vi "Integral.vi"(0 "KIT-QA in":refnum<class "KIT-QA.lvclass">, 1 "-t1":dbl[unit], 2 "t100":dbl[unit], 5 "error in (no error)":errorcluster) -> (14 "KIT-QA out":refnum<class "KIT-QA.lvclass">, 15 "Integral":dbl, 17 "Temperature":dbl, 18 "DCCT@-t1":dbl format="%0.2f", 19 "error out":errorcluster)   [LabVIEW 2015, in "KIT-QA.lvlib" / "KIT-QA.lvclass"]
doc: "Piotr's Integral"
uses:
  KIT-QA.lvclass
  KIT-QA.lvclass/KIT-QA.ctl
  <vilib>/Waveform/WDTOps.llb/WDT Get Waveform Subset DBL.vi
  <vilib>/Waveform/WDTOps.llb/WDT Get XY Value DBL.vi
  <vilib>/Analysis/NI_AALPro.lvlib
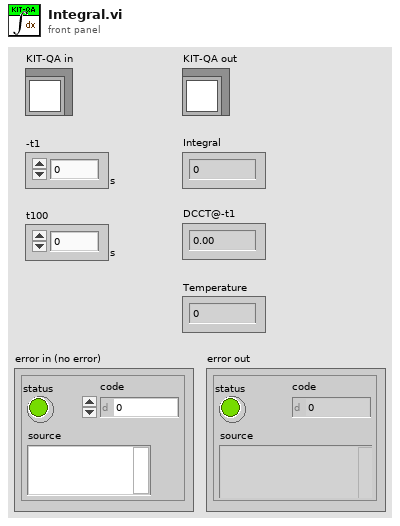
[diagram p1: front panel]
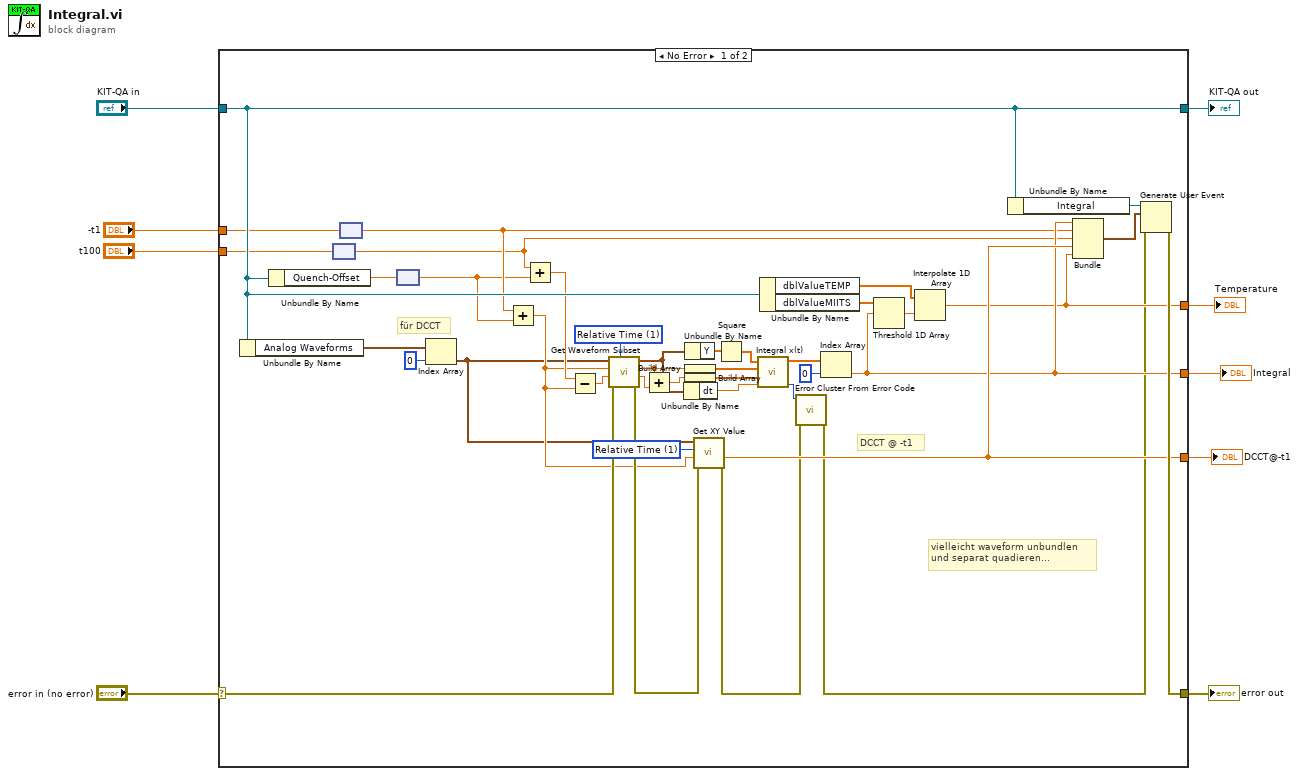
[diagram p0: block diagram]
diagram:
  n1 = case shown="No Error" "error in (no error)" {
    selector: "error in (no error)" -> [w47 w51]
    tunnel: [w49 w51] -> w8
    tunnel: [w31 w50] -> w6
    tunnel: "KIT-QA in" -> [w31 w50]
    tunnel: [w33 _] -> w5
    tunnel: "-t1" -> [w28 _]
    tunnel: "t100" -> [w26 _]
    tunnel: [w41 _] -> w2
    tunnel: [w32 _] -> w1
    frame No Error {
      w10 = u16 1 items=["Samples", "Relative Time"] ("start/duration format")
      w43 = u16 1 items=["Samples", "Relative Time"] ("Y position format")
      # "vielleicht waveform unbundlen\nund separat quadieren..."
      # "DCCT @ -t1"
      # "für DCCT"
      n2 = Unbundle By Name(w31) -> ("Analog Waveforms"=w37:waveform(dbl)[])
      n3 = Unbundle By Name(w31) -> ("Quench-Offset"=w24:dbl[unit])
      n4 = node(w26) -> (w25:dbl)
      n5 = node(w28) -> (w27:dbl)
      n6 = node(w24) -> (w23:dbl)
      n7 = Index Array(array=w37, index=0) -> (element=w17:waveform(dbl))
      n8 = Add(x=w27, y=w23) -> (x+y=w29:dbl)
      n9 = Add(x=w25, y=w23) -> (x+y=w30:dbl)
      n10 = Subtract(x=w30, y=w29) -> (x-y=w39:dbl)
      n11 = call-poly <vilib>:"Get Waveform Subset.vi"("start/duration format"=w10, "error in (no error)"=w47, "duration"=w39, "start samples/time"=w29, "waveform in"=w17) -> ("error out"=w42:errorcluster, "actual duration"=w14:dbl, "actual start samples/time"=w13:dbl, "waveform out"=w16:waveform(dbl))  [unwired: 1 in]
      n12 = Add(x=w13, y=w14) -> (x+y=w12:dbl)
      n13 = Unbundle By Name(w16) -> ("dt"=w44:dbl)
      n14 = Unbundle By Name(w16) -> ("Y"=w19:dbl[])
      n15 = Build Array(w13) -> (w15:dbl[])
      n16 = Build Array(w12) -> (w11:dbl[])
      n17 = call-poly <vilib>:"Get XY Value.vi"("error in (no error)"=w42, "Y position"=w29, "Y position format"=w43, "waveform in"=w17) -> ("error out"=w21:errorcluster, "Y value"=w41:dbl)  [unwired: 3 in, 3 out]
      n18 = Square(x=w19) -> (x^2=w18:dbl[])
      n19 = call <vilib>:"Integral x(t).vi"("dt"=w44, "Final Condition"=w11, "Initial Condition"=w15, "X"=w18) -> ("error"=w22:i32, "Integral X"=w46:dbl[])  [unwired: 6 in]
      n20 = Unbundle By Name(w31) -> ("dblValueTEMP"=w35:dbl[], "dblValueMIITS"=w34:dbl[])
      n21 = call <vilib>:"Error Cluster From Error Code.vi"("error in (no error)"=w21, "error code (0)"=w22) -> ("error out"=w20:errorcluster)  [unwired: 7 in]
      n22 = Index Array(array=w46, index=0) -> (element=w33:dbl)
      n23 = Threshold 1D Array(2:w33, 3:w34) -> (0:w36:dbl)  [unwired: 1 in]
      n24 = Interpolate 1D Array(1:w36, 2:w35) -> (0:w32:dbl)
      n25 = Unbundle By Name(w31) -> ("Integral"=w40:refnum<user-event>)
      n26 = Bundle(w33, w27, w25, "Y value"=w41, w32) -> (w38:cluster{dbl, dbl, dbl, "Y value":dbl, dbl})  [unwired: 1 in]
      n27 = Generate User Event(user event=w40, event data cluster=w38, error in=w20) -> (error out=w49:errorcluster)  [unwired: 1 in, 1 out]
    }
    frame Error {
    }
  }
  "error out" <- w8
  "KIT-QA out" <- w6
  "Integral" <- w5
  "DCCT@-t1" <- w2
  "Temperature" <- w1
